vi "Close.vi"(8 "error in (no error)":errorcluster, 11 "TalonDrive in":refnum<class "TalonDrive.lvclass">) -> (0 "error out":errorcluster, 3 "TalonDrive out":refnum<class "TalonDrive.lvclass">)   [LabVIEW 2017, in "Drive.lvlib" / "TalonDrive.lvclass"]
uses:
  TalonDrive.lvclass
  Drive.lvclass
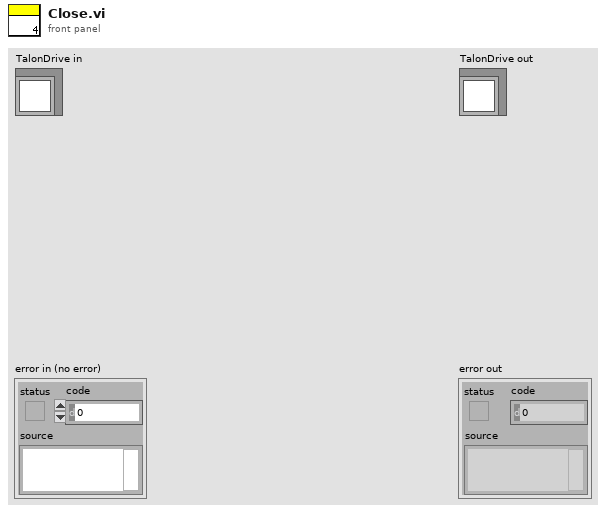
[diagram p1: front panel]
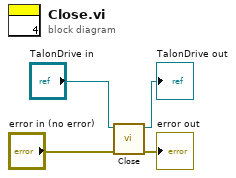
[diagram p0: block diagram]
diagram:
  n1 = call-parent "Close.vi"("error in (no error)"="error in (no error)", "Drive in"="TalonDrive in") -> ("error out"=→"error out":errorcluster, "Drive out"=→"TalonDrive out":refnum<class "TalonDrive.lvclass">)  [unwired: 8 in]
